vi "manual_controller.vi"() -> ()   [LabVIEW 2010]
uses:
  MagiQmw3.lvclass
panel:
  out "Updates":i32
  in  "Slot":u16=4 max=10
  in  "Clock type":enum8{"Internal", "External", "PXI"}(ring)
  in  "ch2 enable":bool
  in  "Ch2 freq":dbl=25.0 caption="Frequency (MHz)" min=25.0 max=6000.0
  in  "Ch2 atten":i32(slide) min=0 max=10 step=1 scale=0.01..10.0
  in  "ch1 enable":bool
  in  "Ch1 freq":dbl=7000.0 caption="Frequency (MHz)" min=7000.0 max=13500.0
  in  "Ch1 atten":i32(slide) min=0 max=10 step=1 scale=0.01..10.0
  in  "stop":bool
  in  "ch0 enable":bool
  in  "Ch0 freq":dbl=25.0 caption="Frequency (MHz)" min=25.0 max=6000.0
  in  "Ch0 atten":i32(slide) min=0 max=10 step=1 scale=0.01..10.0
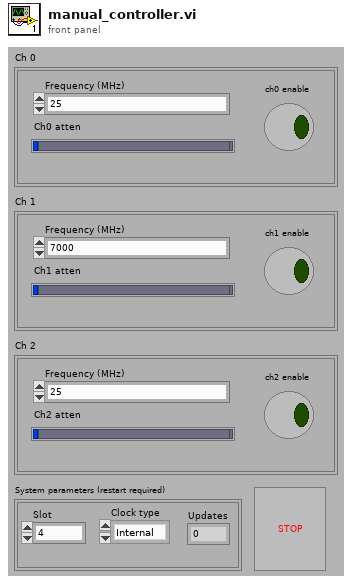
[diagram p1: front panel]
types:
  T1 = cluster{"ch0 enable":bool, "Ch0 freq":dbl, "Ch0 atten":i32}
  T2 = cluster{"ch1 enable":bool, "Ch1 freq":dbl, "Ch1 atten":i32}
  T3 = cluster{"ch2 enable":bool, "Ch2 freq":dbl, "Ch2 atten":i32}
  T4 = cluster{"ch2 enable":bool, "Ch2 freq":dbl, "Ch2 atten":i32}[]
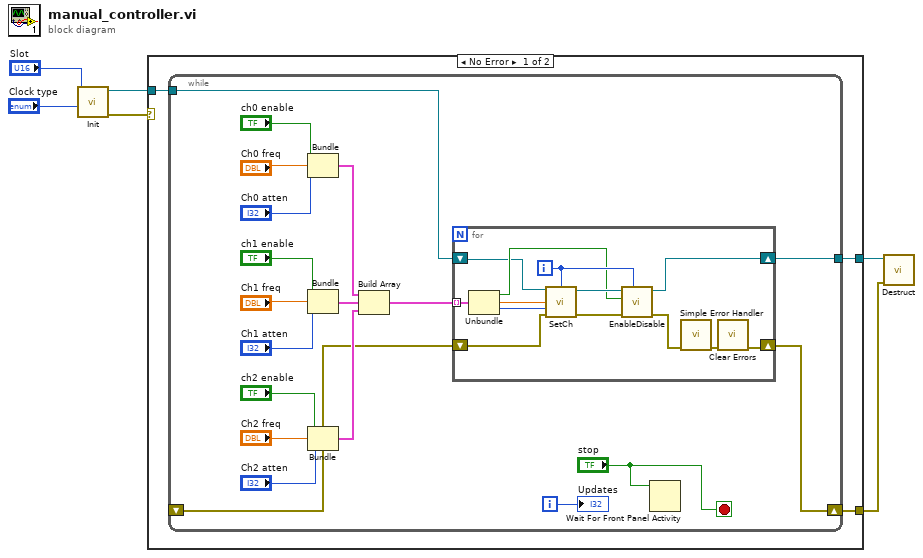
[diagram p0: block diagram]
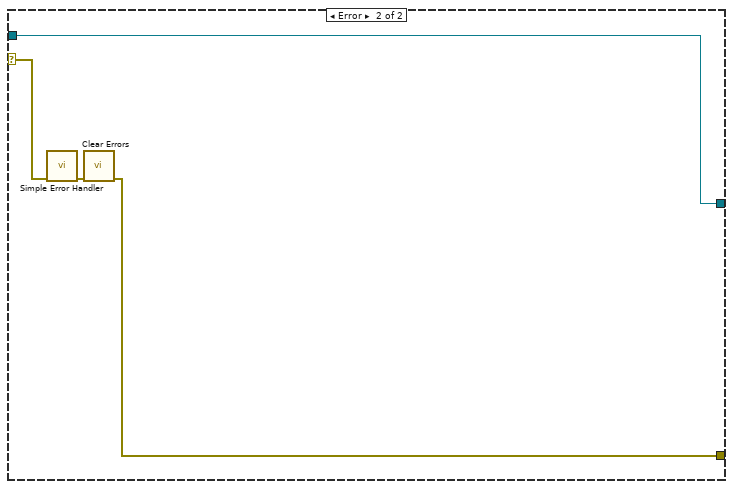
[diagram p2: hidden frame]
diagram:
  n1 = call "Init.vi"("Clock type"="Clock type", "Slot"="Slot") -> ("error out"=w1:errorcluster, "MagiQmw3 out"=w6:refnum<class "MagiQmw3.lvclass">)  [unwired: 8 in]
  n2 = case shown="No Error" w1 {
    selector: w1 -> [_ w44]
    tunnel: w6 -> [w9 w42]
    tunnel: [w8 w42] -> w3
    tunnel: [w7 w43] -> w2
    frame No Error {
      n3 = while {
        tunnel: w9 -> [w11]
        tunnel: [w15] -> w8
        shift-right: [w13] -> w7
        shift-left: _ -> [w12]
        i -> [w10]
        stop <- "stop" stop-if-true
        n4 = Bundle("ch0 enable"="ch0 enable", "Ch0 freq"="Ch0 freq", "Ch0 atten"="Ch0 atten") -> (w19:T1)  [unwired: 1 in]
        n5 = Bundle("ch1 enable"="ch1 enable", "Ch1 freq"="Ch1 freq", "Ch1 atten"="Ch1 atten") -> (w18:T2)  [unwired: 1 in]
        n6 = Bundle("ch2 enable"="ch2 enable", "Ch2 freq"="Ch2 freq", "Ch2 atten"="Ch2 atten") -> (w17:T3)  [unwired: 1 in]
        n7 = Build Array(w19, w18, w17) -> (w16:T4)
        n8 = for {
          tunnel: w16 -> [w41] mode=indexing
          shift-right: [w31] -> w13
          shift-left: w12 -> [w34]
          shift-right: [w33] -> w15
          shift-left: w11 -> [w29]
          i -> [w38]
          n9 = Unbundle(w41) -> ("ch2 enable"=w37:bool, "Ch2 freq"=w36:dbl, "Ch2 atten"=w35:i32)
          n10 = call "SetCh.vi"("MagiQmw3 in"=w29, "ch"=w38, "freq"=w36, "atten"=w35, "error in (no error)"=w34) -> ("MagiQmw3 out"=w40:refnum<class "MagiQmw3.lvclass">, "error out"=w39:errorcluster)  [unwired: 9 in]
          n11 = call "EnableDisable.vi"("ch"=w38, "error in (no error)"=w39, "Enable"=w37, "MagiQmw3 in"=w40) -> ("error out"=w30:errorcluster, "MagiQmw3 out"=w33:refnum<class "MagiQmw3.lvclass">)  [unwired: 6 in]
          n12 = call <vilib>:"Simple Error Handler.vi"("error in (no error)"=w30) -> ("error out"=w32:errorcluster)  [unwired: 4 in, 4 out]
          n13 = call <vilib>:"Clear Errors.vi"("error in (no error)"=w32) -> ("error out"=w31:errorcluster)  [unwired: 6 in]
        }
        n14 = Wait For Front Panel Activity(3:"stop") -> ()  [unwired: 2 in, 1 out]
        "Updates" <- w10
      }
    }
    frame Error {
      n15 = call <vilib>:"Simple Error Handler.vi"("error in (no error)"=w44) -> ("error out"=w45:errorcluster)  [unwired: 4 in, 4 out]
      n16 = call <vilib>:"Clear Errors.vi"("error in (no error)"=w45) -> ("error out"=w43:errorcluster)  [unwired: 6 in]
    }
  }
  n17 = call "Destruct.vi"("error in (no error)"=w2, "MagiQmw3 in"=w3) -> ()  [unwired: 9 in, 1 out]
